vi "get and check open config.vi"(9 "App Name":string, 11 "Working Directory In":path) -> (0 "error out":errorcluster, 1 "ConnectionType":string="LJM_ctANY", 2 "DeviceType":string="LJM_dtANY", 3 "Working Directory Out":path, 4 "Identifier":string="LJM_idANY", 6 "Device Open Config File Name":string)   [LabVIEW 2020]
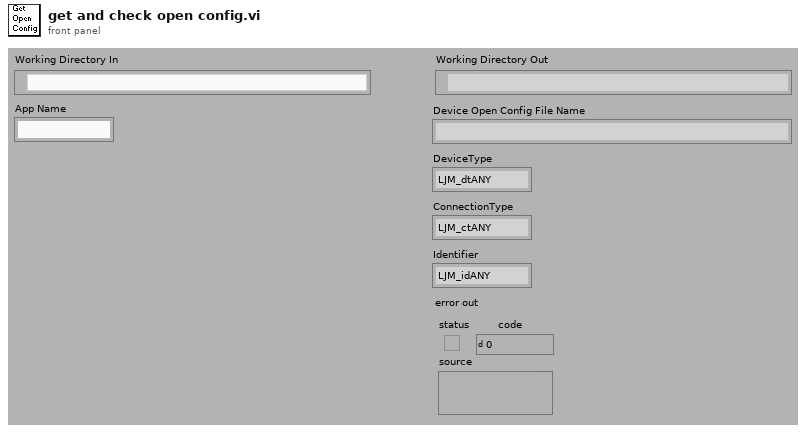
[diagram p1: front panel]
types:
  T1 = enum16{"Left Button", "Center Button", "Right Button", "Window Close"}
  T2 = enum32{"existing file", "new file", "new or existing file", "existing dir", "new dir", "new or existing dir", "existing file (use LLBs)", "new file (use LLBs)", "new or existing file (use LLBs)", "new or existing file or directory (use LLBs)"}
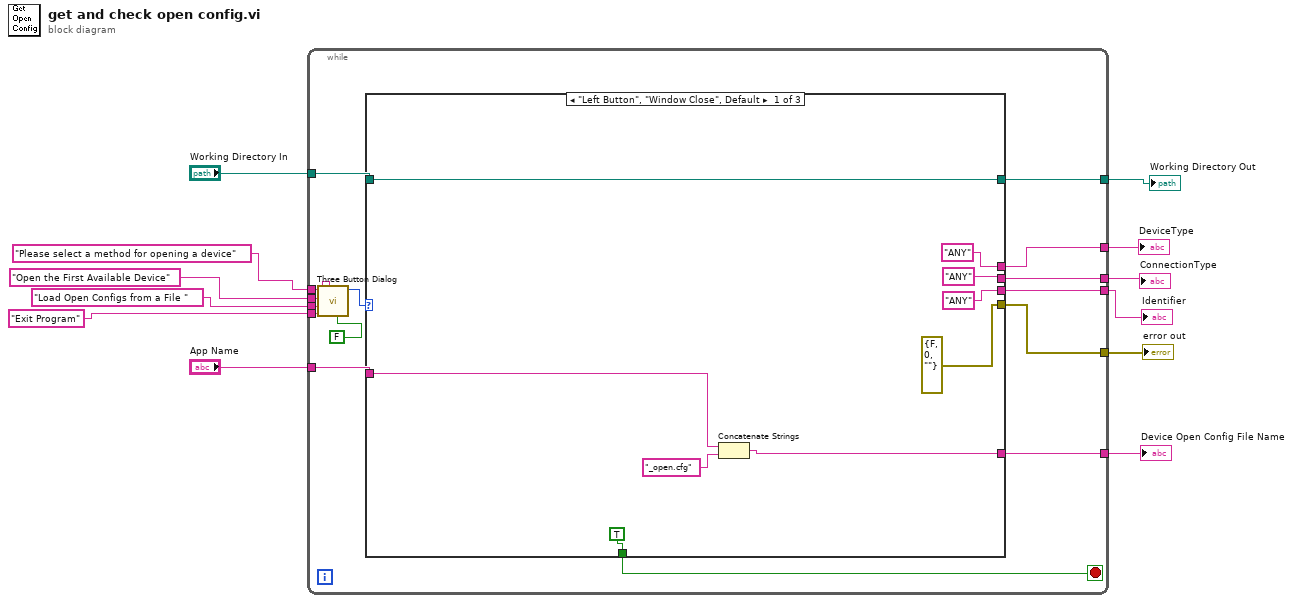
[diagram p0: block diagram]
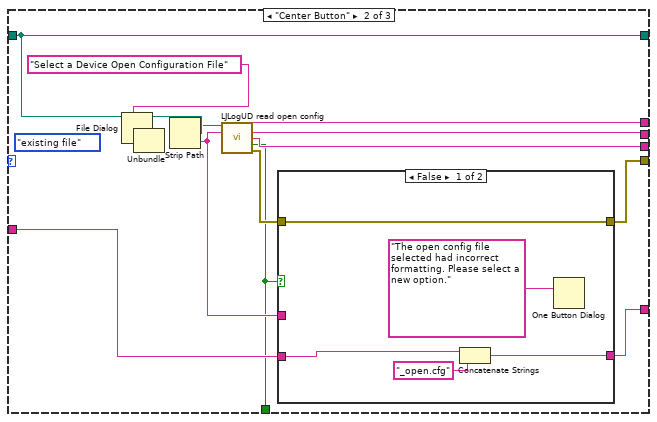
[diagram p2: hidden frame]
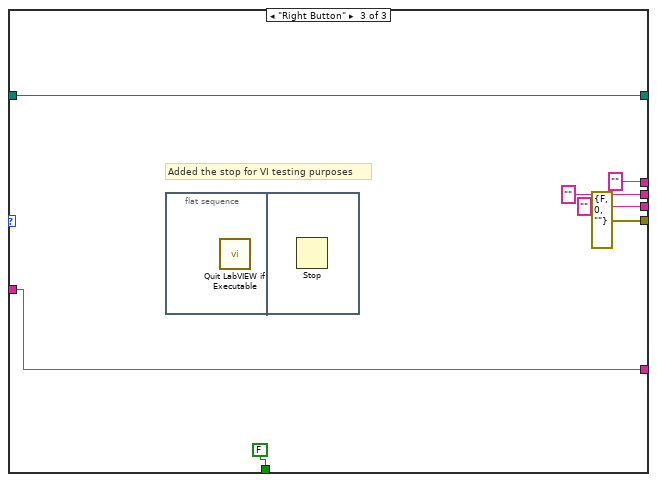
[diagram p4: hidden frame]
diagram:
  n1 = while {
    tunnel: "Working Directory In" -> [w27]
    tunnel: [w26] -> w11
    tunnel: "App Name" -> [w25]
    tunnel: [w24] -> w9
    tunnel: [w23] -> w8
    tunnel: [w22] -> w7
    tunnel: [w21] -> w6
    tunnel: [w20] -> w5
    tunnel: "Please select a method for opening a device" ("message") -> [w14]
    tunnel: "Open the First Available Device" ("F button name (\"Cancel\")") -> [w17]
    tunnel: "Load Open Configs from a File " ("T button name (\"OK\")") -> [w16]
    tunnel: "Exit Program" ("Right Button Text (\"Cancel\")") -> [w15]
    stop <- w19 stop-if-true
    n2 = call <vilib>:"Three Button Dialog.vi"("Allow user to close window? (TRUE)"=FALSE, "Window Title (\"\")"=w14, "Right Button Text (\"Cancel\")"=w15, "Center Button Text (\"No\")"=w16, "Left Button Text (\"Yes\")"=w17, "message"=w14) -> ("Which Button?"=w18:T1)  [unwired: 5 in]
    n3 = case shown="\"Left Button\", \"Window Close\", Default" w18 {
      tunnel: w27 -> [w33 w41 w58]
      tunnel: [w34 w45 w63] -> w26
      tunnel: w25 -> [w35 w46 w63]
      tunnel: [errorcluster {"status"=FALSE, "code"=0, "source"=""} ("error out") w42 errorcluster {"status"=FALSE, "code"=0, "source"=""} ("error out")] -> w24
      tunnel: ["ANY" w49 "" ("Identifier")] -> w23
      tunnel: ["ANY" w48 "" ("ConnectionType")] -> w22
      tunnel: ["ANY" w47 "" ("DeviceType")] -> w21
      tunnel: [w33 w41 w58] -> w20
      tunnel: [TRUE ("Good Open Config") w38 FALSE ("Good Open Config")] -> w19
      frame "Left Button", "Window Close", Default {
        n4 = Concatenate Strings(w35, "_open.cfg" ("filename")) -> (w34:string)
      }
      frame "Center Button" {
        (unwired) T2."existing file" ("select mode (2)")
        n5 = File Dialog(7:"Select a Device Open Configuration File" ("Substring"), 11:w41) -> (0:w37:errorcluster, 3:w44:path)  [unwired: 5 in, 2 out]
        n6 = Unbundle(w37) -> ()  [unwired: 3 out]
        n7 = Strip Path(path=w44) -> (stripped path=w40:path, name=w39:string)
        n8 = call "LJLogUD read open config.vi"("Working Directory"=w40, "filename"=w39) -> ("DeviceType"=w47:string, "ConnectionType"=w48:string, "Identifier"=w49:string, "Good Open Config"=w38:bool, "error out"=w43:errorcluster)  [unwired: 9 in]
        n9 = case shown="False" w38 {
          tunnel: w46 -> [w53 _]
          tunnel: [w52 w57] -> w45
          tunnel: w39 -> [_ w57]
          tunnel: w43 -> [w51 w56]
          tunnel: [w51 w56] -> w42
          frame False {
            n10 = Concatenate Strings(w53, "_open.cfg" ("string")) -> (w52:string)
            n11 = One Button Dialog(message="The open config file selected had incorrect formatting. Please select a new option.") -> ()  [unwired: 1 in, 1 out]
          }
          frame True {
          }
        }
      }
      frame "Right Button" {
        # "Added the stop for VI testing purposes"
        n12 = flat-sequence {
          frame #0 {
            n13 = call "Quit LabVIEW if Executable.vi"() -> ()  [unwired: 1 in]
          }
          frame #1 {
            n14 = Stop() -> ()  [unwired: 1 in]
          }
        }
      }
    }
  }
  "Device Open Config File Name" <- w11
  "DeviceType" <- w6
  "ConnectionType" <- w7
  "Identifier" <- w8
  "error out" <- w9
  "Working Directory Out" <- w5
